vi "Kinect.vi"(8 "Right Right / Left 2":refnum<vi>, 9 "Right Up / Down 2":refnum<vi>, 10 "Left Right / Left 2":refnum<vi>, 11 "Left Up / Down 2":refnum<vi>) -> ()   [LabVIEW 2014]
doc: "Use this template to build a producer/consumer design pattern with events to produce queue items. Use this design pattern instead of the User Interface Event Handler pattern for user interfaces when you want to execute code asynchronously in response to an event without slowing the user interface responsiveness."
uses:
  System.Speech
  Kinect Library/Kinect Type Defs/Color Image Format.ctl
  Kinect Library/Kinect Type Defs/Depth Image Format.ctl
  Kinect Library/Kinect Session Class/Kinect Session.lvclass
  Kinect Library/Kinect Library.lvlib
panel:
  out "Start / Stop":bool
  out "Left Right / Left":sgl(slide) min=-0.5 max=0.5 scale=0.5..-0.5
  out "Right Right / Left":sgl(slide) min=-0.5 max=0.5 scale=-0.5..0.5
  out "Right Up / Down":sgl(slide) min=-0.5 max=0.5 scale=-0.5..0.5
  out "Left Up / Down":sgl(slide) min=-0.5 max=0.5 scale=-0.5..0.5
  out "Skeletal Data":T1(array[cluster])
  in  "Kinect\nVertical Angle\n[Enter]":i32(slide) min=-27 max=27 scale=-27.0..27.0
  out "Depth Frame":T2(plugin-control)
  out "Color Frame":T2(plugin-control)
  out "Status":string="Disconnected"
  in  "Disconnect Button":bool
  in  "Connect Kinect":bool
  in  "stop":bool
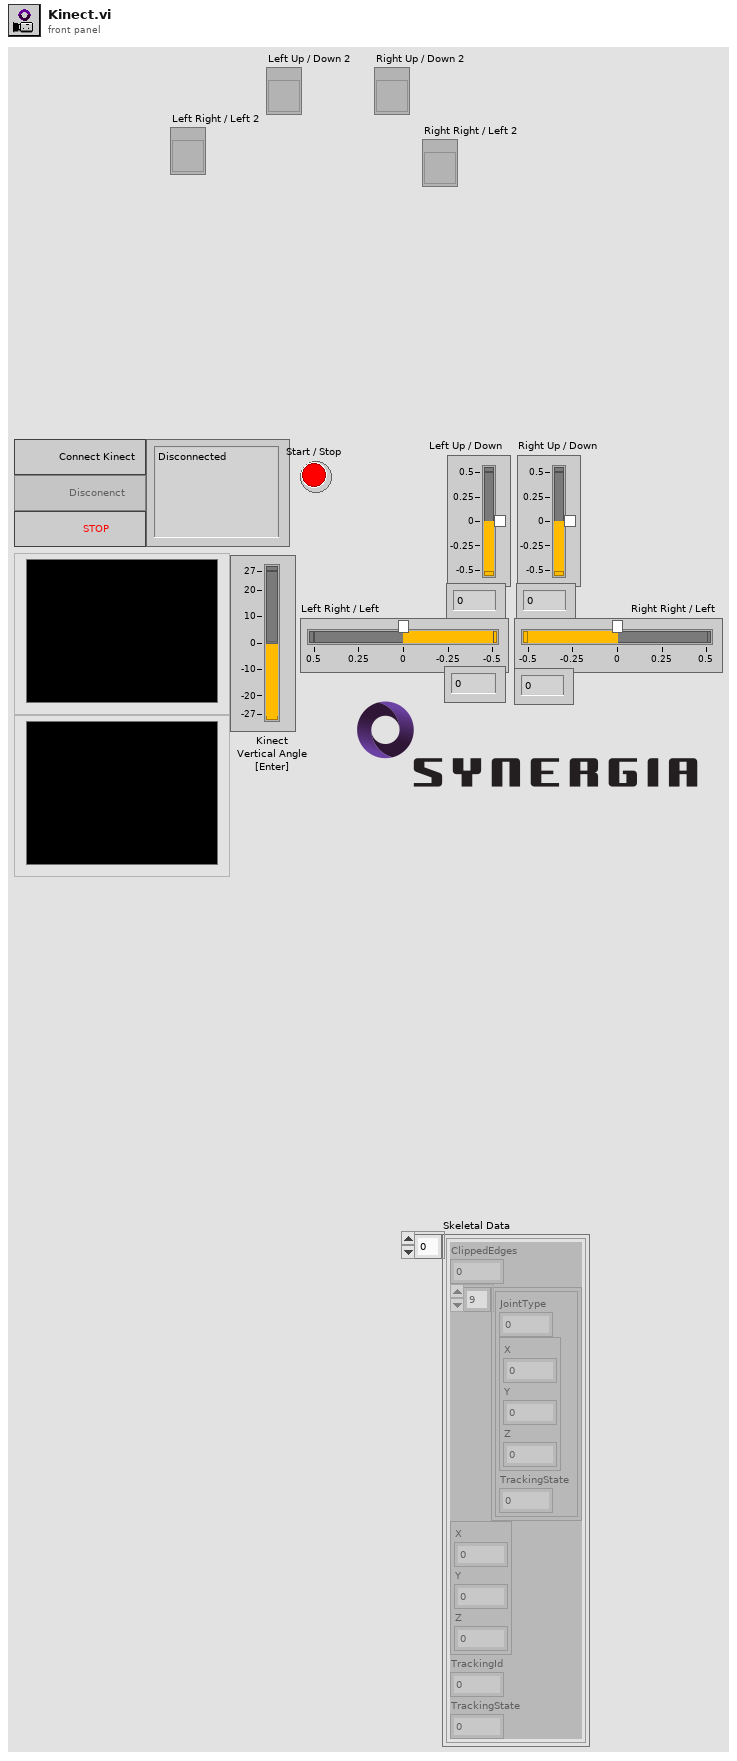
[diagram p1: front panel]
types:
  T1 = cluster{"ClippedEdges":i32, cluster{"JointType":i32, cluster{"X":sgl, "Y":sgl, "Z":sgl}, "TrackingState":i32}[], cluster{"X":sgl, "Y":sgl, "Z":sgl}, "TrackingId":i32, "TrackingState":i32}[]
  T2 = typedef "IMAQ Image.ctl" = refnum<image>
  T3 = enum8{"Enabled", "Disabled", "Disabled and Grayed Out"}
  T4 = typedef "Kinect Library.lvlib/Depth Image Format.ctl" = enum16{"Default", "Undefined", "Resolution640x480Fps30", "Resolution320x240Fps30", "Resolution80x60Fps30"}
  T5 = typedef "Kinect Library.lvlib/Color Image Format.ctl" = enum16{"Default", "Undefined", "RgbResolution640x480Fps30", "RgbResolution1280x960Fps12", "YuvResolution640x480Fps15", "RawYuvResolution640x480Fps15"}
  T6 = cluster{"ClippedEdges":i32, cluster{"JointType":i32, cluster{"X":sgl, "Y":sgl, "Z":sgl}, "TrackingState":i32}[], cluster{"X":sgl, "Y":sgl, "Z":sgl}, "TrackingId":i32, "TrackingState":i32}
  T7 = cluster{"JointType":i32, cluster{"X":sgl, "Y":sgl, "Z":sgl}, "TrackingState":i32}[]
  T8 = cluster{"JointType":i32, cluster{"X":sgl, "Y":sgl, "Z":sgl}, "TrackingState":i32}
  T9 = typedef "eventvkey.ctl" = enum16{"ASCII", "Enter", "Return", "Shift", "Ctrl", "Alt", "Cmd", "Opt", "Caps", "NumLock", "Clear", "Break", "Up", "Down", "Left", "Right", "Insert", "Delete", "Home", "End", "PageUp", "PageDown", "Escape", "Help", "Pause", "ScrollLock", "F1", "F2", "F3", "F4", "F5", "F6", "F7", "F8", "F9", "F10", "F11", "F12", "F13", "F14", "F15", "F16", "F17", "F18", "F19", "F20", "F21", "F22", "F23", "F24", "Play", "VolumeUp", "VolumeDown", "Mute", "Two Byte Char"}
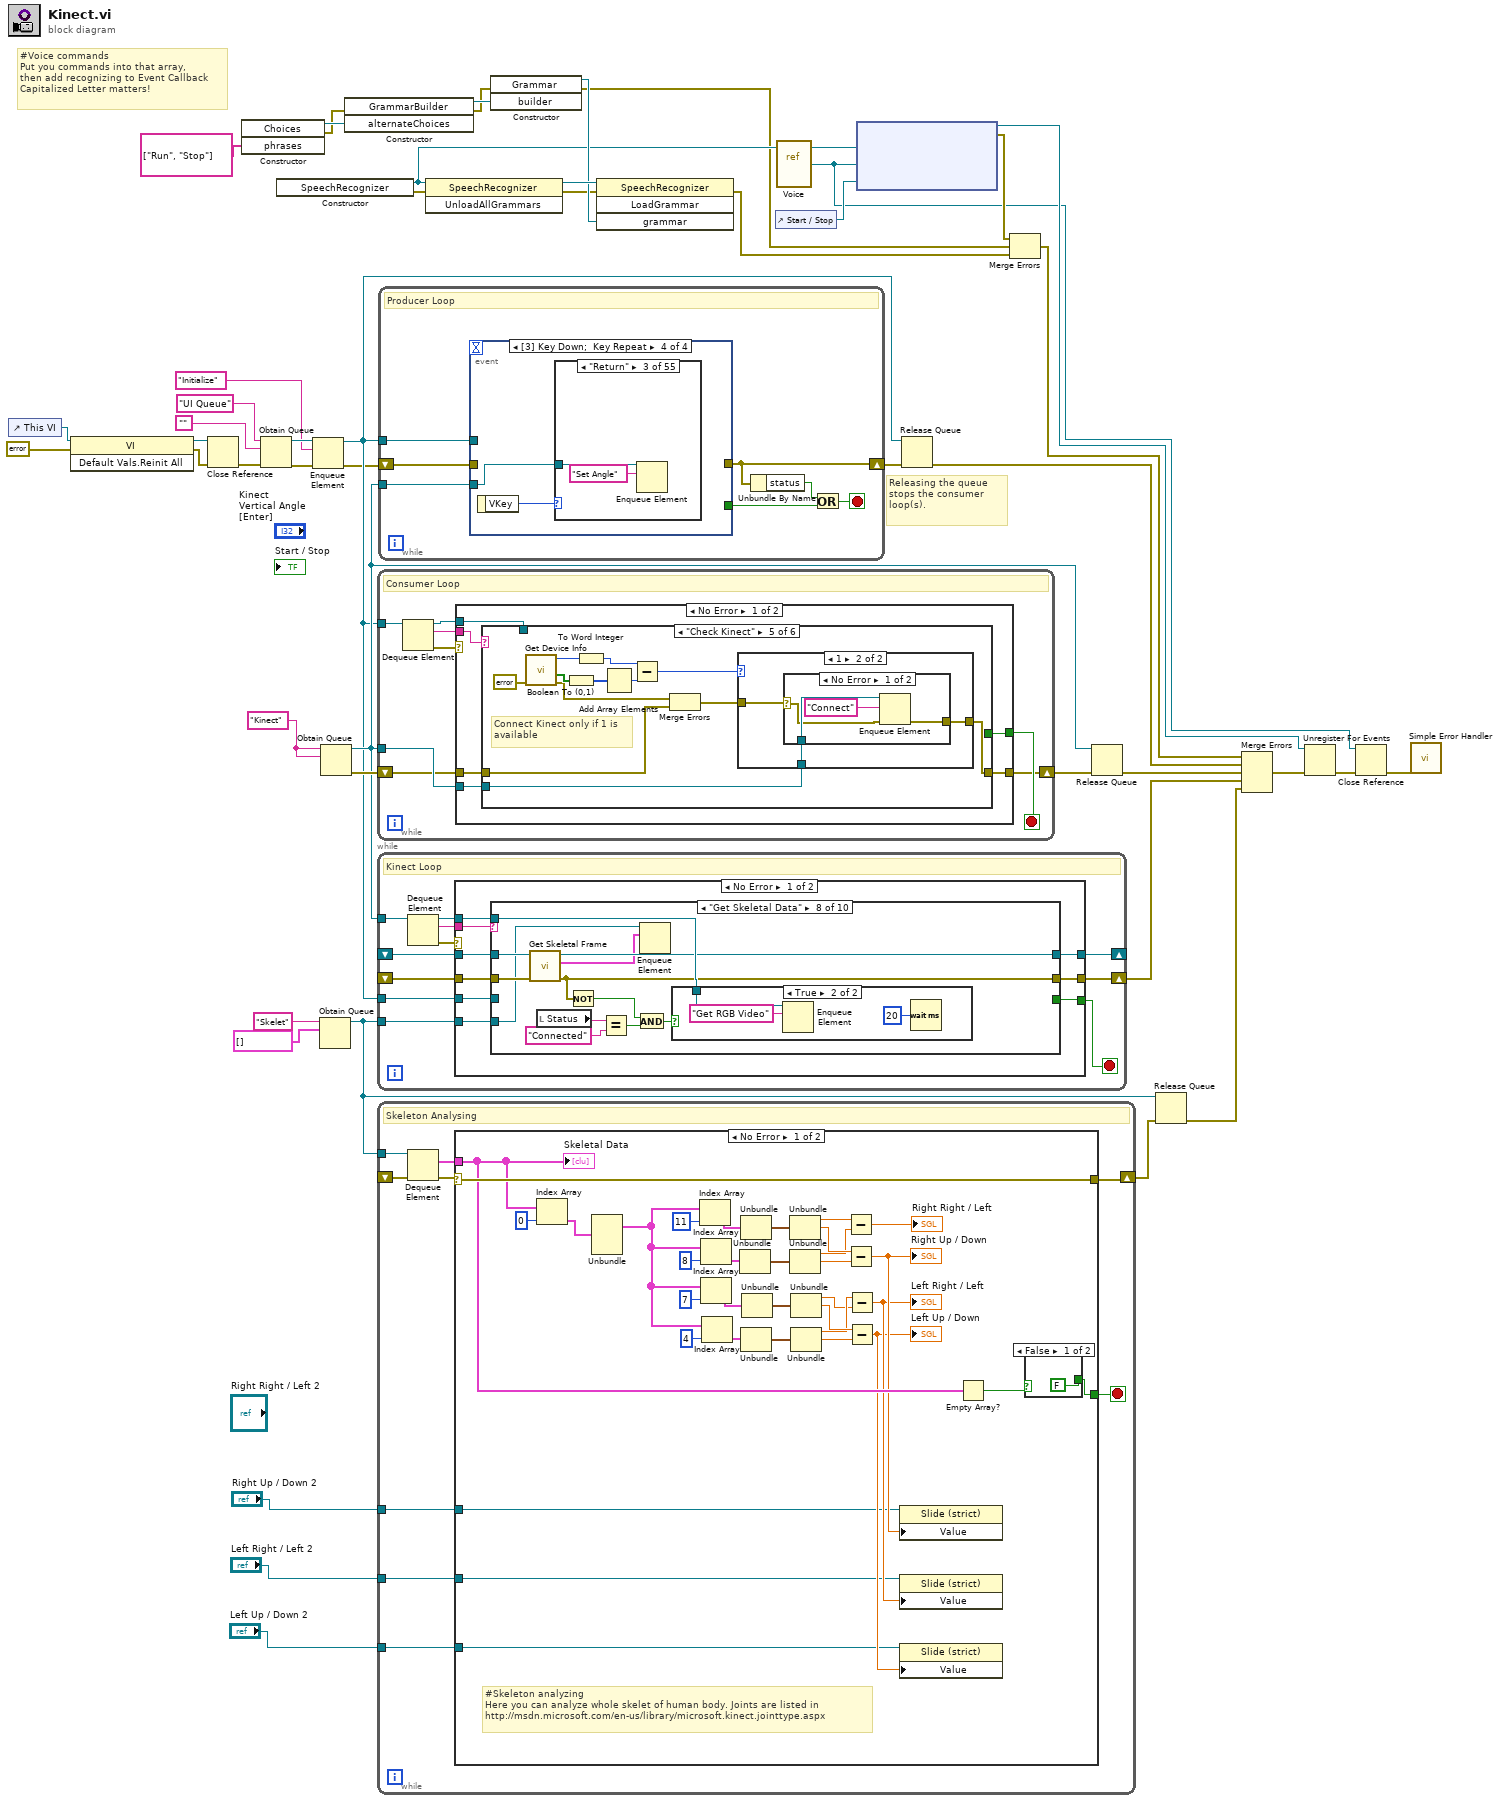
[diagram p0: block diagram]
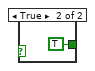
[diagram p2: hidden frame]
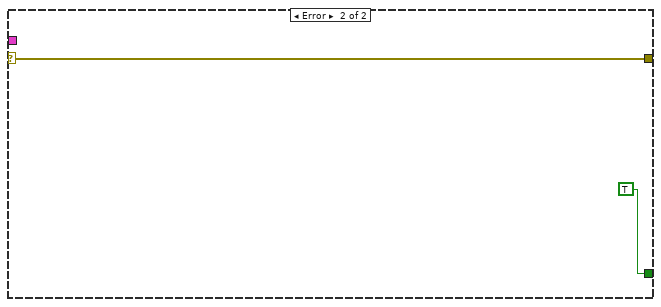
[diagram p3: hidden frame]
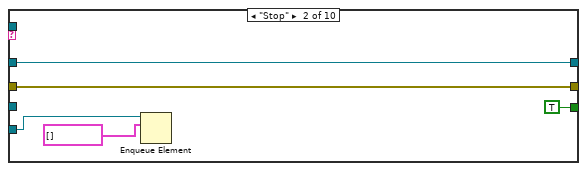
[diagram p5: hidden frame]
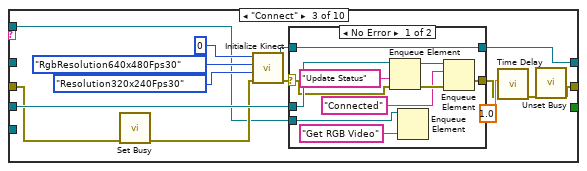
[diagram p6: hidden frame]
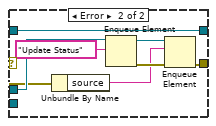
[diagram p7: hidden frame]
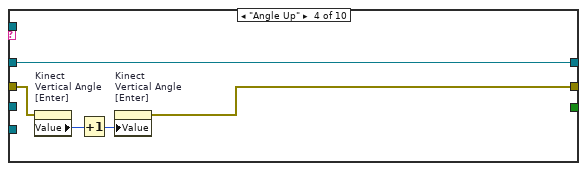
[diagram p8: hidden frame]
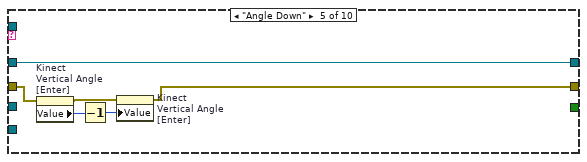
[diagram p9: hidden frame]
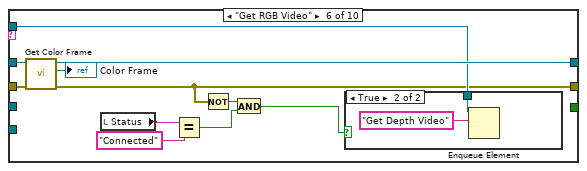
[diagram p10: hidden frame]
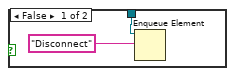
[diagram p11: hidden frame]
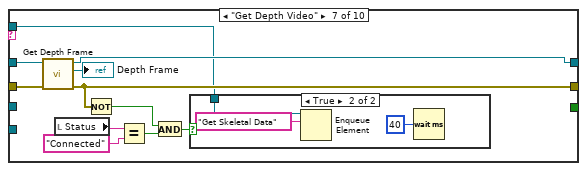
[diagram p12: hidden frame]
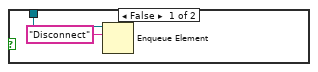
[diagram p13: hidden frame]
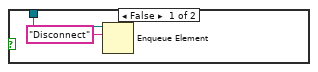
[diagram p14: hidden frame]
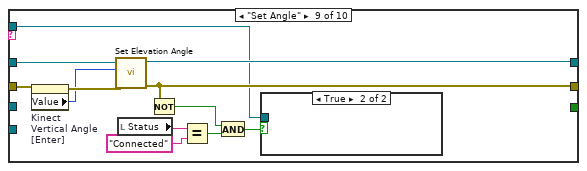
[diagram p15: hidden frame]
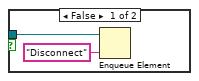
[diagram p16: hidden frame]
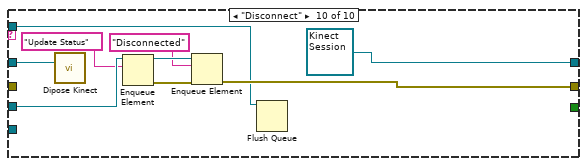
[diagram p17: hidden frame]
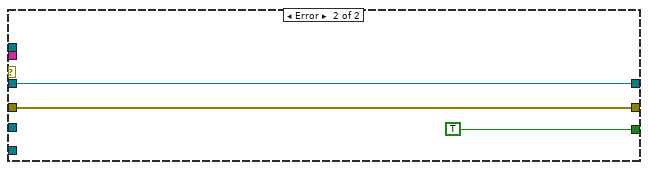
[diagram p18: hidden frame]
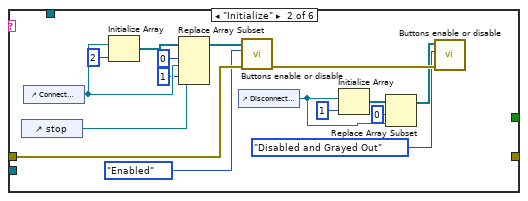
[diagram p20: hidden frame]
diagram:
  w38 = "Kinect" ("name (unnamed)")
  # "#Voice commands\nPut you commands into that array,\nthen add recognizing to Event Callback\nCapitalized Letter matters!"
  # "Releasing the queue stops the consumer loop(s)."
  n1 = control-ref of="This VI"() -> (w45:refnum<vi>)
  n2 = invoke class="VI" method="Default Vals.Reinit All"(reference=w45, error in=errorcluster {"status"=FALSE, "code"=0, "source"=""} ("error in (no error)")) -> (reference out=w44:refnum<vi>, error out=w43:errorcluster)  [unwired: 1 in, 1 out]
  n3 = Close Reference(reference=w44, error in (no error)=w43) -> (error out=w42:errorcluster)
  n4 = constructor class="Choices"("phrases"=string[] ["Run", "Stop"]) -> (reference out=w22:refnum<k24>, error out=w16:errorcluster)  [unwired: 3 in, 2 out]
  n5 = Obtain Queue(name (unnamed)="UI Queue", element data type="" ("data (can be any type)"), error in (no error)=w42) -> (queue out=w33:refnum<queue>, error out=w30:errorcluster)  [unwired: 2 in, 1 out]
  n6 = constructor class="SpeechRecognizer"() -> (reference out=w18:refnum<k24>, error out=w14:errorcluster)  [unwired: 3 in, 1 out]
  n7 = Enqueue Element(queue=w33, element="Initialize", error in (no error)=w30) -> (queue out=w32:refnum<queue>, error out=w31:errorcluster)  [unwired: 1 in, 1 out]
  n8 = Obtain Queue(name (unnamed)="Skelet", element data type=T1 [] ("Skeletal Data")) -> (queue out=w25:refnum<queue>)  [unwired: 3 in, 2 out]
  n9 = Obtain Queue(name (unnamed)=w38, element data type=w38) -> (queue out=w34:refnum<queue>, error out=w40:errorcluster)  [unwired: 3 in, 1 out]
  n10 = constructor class="GrammarBuilder"(error in=w16, "alternateChoices"=w22) -> (reference out=w21:refnum<k24>, error out=w15:errorcluster)  [unwired: 2 in, 2 out]
  n11 = while {
    tunnel: w32 -> [w56]
    shift-right: [w51] -> w39
    shift-left: w40 -> [w50]
    tunnel: w34 -> [w52]
    stop <- w53 stop-if-true
    # "Consumer Loop"
    n12 = Dequeue Element(queue=w56) -> (queue out=w49:refnum<queue>, element=w54:string, error out=w55:errorcluster)  [unwired: 2 in, 1 out]
    n13 = case shown="No Error" w55 {
      selector: w55 -> [_ w136]
      tunnel: w54 -> [w62 _]
      tunnel: [w57 TRUE] -> w53
      tunnel: w52 -> [w61 _]
      tunnel: [w60 w136] -> w51
      tunnel: w50 -> [w59 _]
      tunnel: w49 -> [w58 _]
      frame No Error {
        n14 = case shown="\"Check Kinect\"" w62 {
          tunnel: w61 -> [_ _ _ _ w113 w135]
          tunnel: [w63 _ w80 w82 w112 w132] -> w60
          tunnel: w59 -> [w63 w73 w80 w85 w110 w133]
          tunnel: w58 -> [_ _ _ w87 _ _]
          tunnel: [_ _ TRUE _ _ _] -> w57
          frame Default {
          }
          frame "Initialize" {
            n15 = control-ref of="stop"() -> (w74:refnum<vi>)
            n16 = control-ref of="Connect Kinect"() -> (w76:refnum<vi>)
            n17 = Initialize Array(w76, 2 ("dimension size")) -> (w78:refnum<vi>[])
            n18 = Replace Array Subset(array=w78, new element #1=w76, index #1=0 ("index"), new element #2=w74, index #2=1 ("index")) -> (w72:refnum<vi>[])
            n19 = control-ref of="Disconnect Button"() -> (w66:refnum<vi>)
            n20 = call "Buttons enable or disable.vi"("error in (no error)"=w73, "Enabled or Disabled?"=T3."Enabled", "Input references array"=w72) -> ("error out"=w70:errorcluster)  [unwired: 8 in]
            n21 = Initialize Array(w66, 1 ("dimension size")) -> (w68:refnum<vi>[])
            n22 = Replace Array Subset(array=w68, new element=w66, index=0) -> (w65:refnum<vi>[])
            n23 = call "Buttons enable or disable.vi"("error in (no error)"=w70, "Enabled or Disabled?"=T3."Disabled and Grayed Out", "Input references array"=w65) -> ()  [unwired: 8 in, 1 out]
          }
          frame "Stop" {
          }
          frame "Update Status" {
            n24 = Dequeue Element(queue=w87) -> (element=w84:string, error out=w86:errorcluster)  [unwired: 2 in, 2 out]
            "Status" <- w84
            n25 = Merge Errors(w86, w85) -> (w83:errorcluster)
            n26 = case shown="\"Disconnected\"" w84 {
              tunnel: w83 -> [w88 w96 w108]
              tunnel: [w88 w90 w99] -> w82
              frame Default {
              }
              frame "Connected" {
                n27 = control-ref of="Disconnect Button"() -> (w98:refnum<vi>)
                n28 = Build Array(w98) -> (w97:refnum<vi>[])
                n29 = call "Buttons enable or disable.vi"("error in (no error)"=w96, "Enabled or Disabled?"=T3."Enabled", "Input references array"=w97) -> ("error out"=w91:errorcluster)  [unwired: 8 in]
                n30 = control-ref of="stop"() -> (w93:refnum<vi>)
                n31 = control-ref of="Connect Kinect"() -> (w92:refnum<vi>)
                n32 = Build Array(w93, w92) -> (w94:refnum<vi>[])
                n33 = call "Buttons enable or disable.vi"("error in (no error)"=w91, "Enabled or Disabled?"=T3."Disabled and Grayed Out", "Input references array"=w94) -> ("error out"=w90:errorcluster)  [unwired: 8 in]
              }
              frame "Disconnected" {
                n34 = control-ref of="Disconnect Button"() -> (w107:refnum<vi>)
                n35 = Build Array(w107) -> (w106:refnum<vi>[])
                n36 = call "Buttons enable or disable.vi"("error in (no error)"=w108, "Enabled or Disabled?"=T3."Disabled and Grayed Out", "Input references array"=w106) -> ("error out"=w101:errorcluster)  [unwired: 8 in]
                n37 = control-ref of="Connect Kinect"() -> (w103:refnum<vi>)
                n38 = control-ref of="stop"() -> (w102:refnum<vi>)
                n39 = Build Array(w103, w102) -> (w104:refnum<vi>[])
                n40 = call "Buttons enable or disable.vi"("error in (no error)"=w101, "Enabled or Disabled?"=T3."Enabled", "Input references array"=w104) -> ("error out"=w99:errorcluster)  [unwired: 8 in]
              }
            }
          }
          frame "Check Kinect" {
            # "Connect Kinect only if 1 is\navailable"
            n41 = call "Get Device Info.vi"("error in (no error)"=errorcluster {"status"=FALSE, "code"=0, "source"=""}) -> ("error out"=w111:errorcluster, "Is Running"=w119:bool[], "Number of Kinects Attached"=w116:i32)  [unwired: 7 in, 1 out]
            n42 = Boolean To (0,1)(Boolean=w119) -> (0, 1=w118:i16[])
            n43 = To Word Integer(number=w116) -> (16bit integer=w115:i16)
            n44 = Add Array Elements(numeric array=w118) -> (sum=w117:i16)
            n45 = Subtract(x=w115, y=w117) -> (x-y=w114:i16)
            n46 = Merge Errors(w111, w110) -> (w109:errorcluster)
            n47 = case shown="1" w114 {
              tunnel: w109 -> [w122 w124]
              tunnel: w113 -> [_ w125]
              tunnel: [w121 w123] -> w112
              frame 0, Default {
                n48 = call "Display Message to User"("error in (no error)"=w122) -> ("error out"=w121:errorcluster)  [unwired: 9 in, 1 out]
              }
              frame 1 {
                n49 = case shown="No Error" w124 {
                  selector: w124 -> [w127 w131]
                  tunnel: w125 -> [w129 _]
                  tunnel: [w126 w130] -> w123
                  frame No Error {
                    n50 = Enqueue Element(queue=w129, element="Connect", error in (no error)=w127) -> (error out=w126:errorcluster)  [unwired: 1 in, 2 out]
                  }
                  frame Error {
                    n51 = call "Display Message to User2"("error in (no error)"=w131) -> ("error out"=w130:errorcluster)  [unwired: 9 in, 1 out]
                  }
                }
              }
            }
          }
          frame "Disconnect Kinect" {
            n52 = Enqueue Element(queue=w135, element="Disconnect", error in (no error)=w133) -> (error out=w132:errorcluster)  [unwired: 1 in, 2 out]
          }
        }
      }
      frame Error {
        # "Return true in any case that should stop the loop."
      }
    }
  }
  n53 = while {
    tunnel: w34 -> [w148]
    shift-right: [w144] -> _
    shift-left: _ -> [w143]
    shift-right: [w142] -> w35
    shift-left: _ -> [w141]
    tunnel: w32 -> [w140]
    tunnel: w25 -> [w138]
    stop <- w139 stop-if-true
    # "Kinect Loop"
    n54 = Dequeue Element(queue=w148) -> (queue out=w146:refnum<queue>, element=w145:string, error out=w147:errorcluster)  [unwired: 2 in, 1 out]
    n55 = case shown="No Error" w147 {
      tunnel: w146 -> [w151 _]
      tunnel: w145 -> [w157 _]
      tunnel: [w150 TRUE] -> w139
      tunnel: [w156 w280] -> w144
      tunnel: w143 -> [w155 w280]
      tunnel: [w154 w279] -> w142
      tunnel: w141 -> [w153 w279]
      tunnel: w140 -> [w152 _]
      tunnel: w138 -> [w149 _]
      frame No Error {
        n56 = case shown="\"Get Skeletal Data\"" w157 {
          tunnel: [w159 w162 w173 w197 w202 w216 w230 w241 w266 refnum<class "Kinect Session.lvclass"> refnum ("Kinect Session out")] -> w156
          tunnel: w155 -> [w159 w162 _ w197 w202 w218 w233 w242 w267 w277]
          tunnel: [w158 w163 w166 w198 w203 w208 w229 w243 w258 w271] -> w154
          tunnel: w153 -> [w158 w163 w172 w200 w207 w217 w232 w244 w265 _]
          tunnel: w152 -> [_ _ w175 _ _ _ _ _ _ w276]
          tunnel: w151 -> [_ _ w169 _ _ w211 w223 w245 w256 w270]
          tunnel: [_ TRUE _ _ _ _ _ _ _ _] -> w150
          tunnel: w149 -> [_ w161 _ _ _ _ _ w240 _ _]
          frame Default {
          }
          frame "Stop" {
            n57 = Enqueue Element(queue=w161, element=T1 [] ("Skeletal Data")) -> ()  [unwired: 2 in, 3 out]
          }
          frame "Connect" {
            n58 = call <vilib>:"Set Busy.vi"("error in (no error)"=w172) -> ("error out"=w171:errorcluster)  [unwired: 9 in, 1 out]
            n59 = call "Initialize Kinect.vi"("error in (no error)"=w171, "Depth Image Format"=Depth_Image_Format."Resolution320x240Fps30", "Color Image Format"=Color_Image_Format."RgbResolution640x480Fps30", "Kinect Sensor Index"=0) -> ("error out"=w170:errorcluster, "Kinect Session out"=w174:refnum<class "Kinect Session.lvclass">)  [unwired: 6 in]
            n60 = case shown="No Error" w170 {
              selector: w170 -> [w186 w191]
              tunnel: w175 -> [w188 w196]
              tunnel: w174 -> [w181 w189]
              tunnel: [w184 w193] -> w165
              tunnel: [w181 w189] -> w173
              tunnel: w169 -> [w180 _]
              frame No Error {
                n61 = Enqueue Element(queue=w188, element="Update Status", error in (no error)=w186) -> (queue out=w182:refnum<queue>, error out=w185:errorcluster)  [unwired: 1 in, 1 out]
                n62 = Enqueue Element(queue=w180, element="Get RGB Video") -> ()  [unwired: 2 in, 3 out]
                n63 = Enqueue Element(queue=w182, element="Connected", error in (no error)=w185) -> (error out=w184:errorcluster)  [unwired: 1 in, 2 out]
              }
              frame Error {
                n64 = Unbundle By Name(w191) -> ("source"=w190:string)
                n65 = Enqueue Element(queue=w196, element="Update Status") -> (queue out=w194:refnum<queue>, error out=w192:errorcluster)  [unwired: 2 in, 1 out]
                n66 = Enqueue Element(queue=w194, element=w190, error in (no error)=w192) -> (error out=w193:errorcluster)  [unwired: 1 in, 2 out]
              }
            }
            n67 = call "Time Delay"("error in (no error)"=w165, "Delay Time (s)"=1.0) -> ("error out"=w167:errorcluster)  [unwired: 9 in]
            n68 = call <vilib>:"Unset Busy.vi"("error in (no error)"=w167) -> ("error out"=w166:errorcluster)  [unwired: 10 in]
          }
          frame "Angle Up" {
            n69 = property on="Kinect\nVertical Angle\n[Enter]" class="Slide (strict)"(error in=w200) -> ("Value"=w201:i32)  [unwired: 1 in, 2 out]
            n70 = Increment(x=w201) -> (x+1=w199:i32)
            n71 = property on="Kinect\nVertical Angle\n[Enter]" class="Slide (strict)"("Value"=w199) -> (error out=w198:errorcluster)  [unwired: 2 in, 1 out]
          }
          frame "Angle Down" {
            n72 = property on="Kinect\nVertical Angle\n[Enter]" class="Slide (strict)"(error in=w207) -> (error out=w205:errorcluster, "Value"=w206:i32)  [unwired: 1 in, 1 out]
            n73 = Decrement(x=w206) -> (x-1=w204:i32)
            n74 = property on="Kinect\nVertical Angle\n[Enter]" class="Slide (strict)"(error in=w205, "Value"=w204) -> (error out=w203:errorcluster)  [unwired: 1 in, 1 out]
          }
          frame "Get RGB Video" {
            n75 = call "Get Color Frame.vi"("error in (no error)"=w217, "Kinect Session in"=w218) -> ("error out"=w208:errorcluster, "Color Frame"=→"Color Frame":T2, "Kinect Session out"=w216:refnum<class "Kinect Session.lvclass">)  [unwired: 7 in]
            n76 = local read "Status"() -> (w214:string)
            n77 = Equal?(x=w214, y="Connected") -> (x = y?=w209:bool)
            n78 = Not(x=w208) -> (.not. x?=w210:bool)
            n79 = And(x=w210, y=w209) -> (x .and. y?=w212:bool)
            n80 = case shown="True" w212 {
              tunnel: w211 -> [w220 w222]
              frame False {
                n81 = Enqueue Element(queue=w220, element="Disconnect") -> ()  [unwired: 2 in, 3 out]
              }
              frame True {
                n82 = Enqueue Element(queue=w222, element="Get Depth Video") -> ()  [unwired: 2 in, 3 out]
              }
            }
          }
          frame "Get Depth Video" {
            n83 = call "Get Depth Frame.vi"("error in (no error)"=w232, "Kinect Session in"=w233) -> ("error out"=w229:errorcluster, "Depth Frame"=→"Depth Frame":T2, "Kinect Session out"=w230:refnum<class "Kinect Session.lvclass">)  [unwired: 7 in]
            n84 = local read "Status"() -> (w228:string)
            n85 = Not(x=w229) -> (.not. x?=w225:bool)
            n86 = Equal?(x=w228, y="Connected") -> (x = y?=w226:bool)
            n87 = And(x=w225, y=w226) -> (x .and. y?=w224:bool)
            n88 = case shown="True" w224 {
              tunnel: w223 -> [w235 w238]
              frame False {
                n89 = Enqueue Element(queue=w235, element="Disconnect") -> ()  [unwired: 2 in, 3 out]
              }
              frame True {
                n90 = Enqueue Element(queue=w238, element="Get Skeletal Data") -> ()  [unwired: 2 in, 3 out]
                n91 = Wait (ms)(milliseconds to wait=u32 40) -> ()  [unwired: 1 out]
              }
            }
          }
          frame "Get Skeletal Data" {
            n92 = call "Get Skeletal Frame.vi"("error in (no error)"=w244, "Kinect Session in"=w242) -> ("error out"=w243:errorcluster, "Skeletal Data"=w239:T1, "Kinect Session out"=w241:refnum<class "Kinect Session.lvclass">)  [unwired: 7 in]
            n93 = local read "Status"() -> (w250:string)
            n94 = Not(x=w243) -> (.not. x?=w247:bool)
            n95 = Equal?(x=w250, y="Connected") -> (x = y?=w248:bool)
            n96 = And(x=w247, y=w248) -> (x .and. y?=w246:bool)
            n97 = Enqueue Element(queue=w240, element=w239) -> ()  [unwired: 2 in, 3 out]
            n98 = case shown="True" w246 {
              tunnel: w245 -> [w252 w255]
              frame False {
                n99 = Enqueue Element(queue=w252, element="Disconnect") -> ()  [unwired: 2 in, 3 out]
              }
              frame True {
                n100 = Enqueue Element(queue=w255, element="Get RGB Video") -> ()  [unwired: 2 in, 3 out]
                n101 = Wait (ms)(milliseconds to wait=u32 20) -> ()  [unwired: 1 out]
              }
            }
          }
          frame "Set Angle" {
            n102 = property on="Kinect\nVertical Angle\n[Enter]" class="Slide (strict)"(error in=w265) -> (error out=w264:errorcluster, "Value"=w263:i32)  [unwired: 1 in, 1 out]
            n103 = call "Set Elevation Angle.vi"("error in (no error)"=w264, "ElevationAngle"=w263, "Kinect Session in"=w267) -> ("error out"=w258:errorcluster, "Kinect Session out"=w266:refnum<class "Kinect Session.lvclass">)  [unwired: 6 in, 1 out]
            n104 = local read "Status"() -> (w262:string)
            n105 = Not(x=w258) -> (.not. x?=w259:bool)
            n106 = Equal?(x=w262, y="Connected") -> (x = y?=w260:bool)
            n107 = And(x=w259, y=w260) -> (x .and. y?=w257:bool)
            n108 = case shown="True" w257 {
              tunnel: w256 -> [w269 _]
              frame False {
                n109 = Enqueue Element(queue=w269, element="Disconnect") -> ()  [unwired: 2 in, 3 out]
              }
              frame True {
              }
            }
          }
          frame "Disconnect" {
            n110 = call "Dipose Kinect.vi"("Kinect Session in"=w277) -> ()  [unwired: 10 in, 1 out]
            n111 = Enqueue Element(queue=w276, element="Update Status") -> (queue out=w274:refnum<queue>, error out=w272:errorcluster)  [unwired: 2 in, 1 out]
            n112 = Enqueue Element(queue=w274, element="Disconnected", error in (no error)=w272) -> (error out=w271:errorcluster)  [unwired: 1 in, 2 out]
            n113 = Flush Queue(queue=w270) -> ()  [unwired: 1 in, 3 out]
          }
        }
      }
      frame Error {
      }
    }
  }
  n114 = while {
    tunnel: w25 -> [w290]
    shift-right: [w285] -> w24
    shift-left: _ -> [w286]
    tunnel: "Left Up / Down 2" -> [w284]
    tunnel: "Left Right / Left 2" -> [w283]
    tunnel: "Right Up / Down 2" -> [w282]
    stop <- w288 stop-if-true
    # "Skeleton Analysing"
    n115 = Dequeue Element(queue=w290, error in (no error)=w286) -> (element=w287:T1, error out=w289:errorcluster)  [unwired: 1 in, 2 out]
    n116 = case shown="No Error" w289 {
      selector: w289 -> [w324 w327]
      tunnel: [w322 TRUE] -> w288
      tunnel: w287 -> [w321 _]
      tunnel: [w324 w327] -> w285
      tunnel: w284 -> [w293 _]
      tunnel: w283 -> [w292 _]
      tunnel: w282 -> [w291 _]
      frame No Error {
        # "#Skeleton analyzing\nHere you can analyze whole skelet of human body. Joints are listed in\nhttp://msdn.microsoft.com/en-us/library/microsoft.kinect.jointtype.aspx"
        n117 = Index Array(array=w321, index=0) -> (element=w319:T6)
        n118 = Unbundle(w319) -> (w300:T7)  [unwired: 4 out]
        n119 = Index Array(array=w300, index=11) -> (element=w316:T8)
        n120 = Index Array(array=w300, index=8) -> (element=w315:T8)
        n121 = Index Array(array=w300, index=7) -> (element=w303:T8)
        n122 = Index Array(array=w300, index=4) -> (element=w304:T8)
        n123 = Unbundle(w315) -> (w313:cluster{"X":sgl, "Y":sgl, "Z":sgl})  [unwired: 2 out]
        n124 = Unbundle(w316) -> (w314:cluster{"X":sgl, "Y":sgl, "Z":sgl})  [unwired: 2 out]
        n125 = Unbundle(w304) -> (w306:cluster{"X":sgl, "Y":sgl, "Z":sgl})  [unwired: 2 out]
        n126 = Unbundle(w303) -> (w305:cluster{"X":sgl, "Y":sgl, "Z":sgl})  [unwired: 2 out]
        n127 = Unbundle(w314) -> ("X"=w310:sgl, "Y"=w312:sgl)  [unwired: 1 out]
        n128 = Unbundle(w313) -> ("X"=w309:sgl, "Y"=w311:sgl)  [unwired: 1 out]
        n129 = Unbundle(w305) -> ("X"=w298:sgl, "Y"=w307:sgl)  [unwired: 1 out]
        n130 = Unbundle(w306) -> ("X"=w299:sgl, "Y"=w308:sgl)  [unwired: 1 out]
        n131 = Subtract(x=w310, y=w309) -> (x-y=→"Right Right / Left":sgl)
        n132 = Subtract(x=w312, y=w311) -> (x-y=w296:sgl)
        "Right Up / Down" <- w296
        n133 = Subtract(x=w299, y=w298) -> (x-y=w295:sgl)
        "Left Right / Left" <- w295
        n134 = Subtract(x=w307, y=w308) -> (x-y=w294:sgl)
        "Left Up / Down" <- w294
        n135 = property class="Slide (strict)"(reference=w291, "Value"=w296) -> ()  [unwired: 1 in, 2 out]
        n136 = property class="Slide (strict)"(reference=w292, "Value"=w295) -> ()  [unwired: 1 in, 2 out]
        n137 = property class="Slide (strict)"(reference=w293, "Value"=w294) -> ()  [unwired: 1 in, 2 out]
        n138 = Empty Array?(array=w321) -> (empty?=w323:bool)
        n139 = case shown="False" w323 {
          tunnel: [FALSE TRUE] -> w322
          frame False {
          }
          frame True {
          }
        }
        "Skeletal Data" <- w321
      }
      frame Error {
      }
    }
  }
  n140 = while {
    shift-right: [w331] -> w48
    shift-left: w31 -> [w334]
    tunnel: w32 -> [w335]
    tunnel: w34 -> [w329]
    stop <- w332 stop-if-true
    # "Producer Loop"
    n141 = event shown="[3] Key Down;  Key Repeat" {
      selector: _ -> [_ _ _ _]
      dyn-events: _ -> [_ _ _ _]
      timeout: _ -> [_ _ _ _]
      tunnel: w335 -> [w339 w345 w347 _]
      tunnel: w334 -> [w340 w343 w349 _]
      tunnel: [w340 w342 w348 _] -> w331
      tunnel: ["stop" _ _ _] -> w333
      tunnel: w329 -> [w337 _ _ w350]
      event "stop": Value Change {
        n142 = event-data() -> ()  [unwired: 1 in, 1 out]
        n143 = Enqueue Element(queue=w339, element="Stop") -> ()  [unwired: 2 in, 3 out]
        n144 = Enqueue Element(queue=w337, element="Stop") -> ()  [unwired: 2 in, 3 out]
      }
      event "Connect Kinect": Value Change {
        n145 = event-data() -> ()  [unwired: 1 in, 1 out]
        n146 = Enqueue Element(queue=w345, element="Check Kinect", error in (no error)=w343) -> (error out=w342:errorcluster)  [unwired: 1 in, 2 out]
      }
      event "Disconnect Button": Value Change {
        n147 = event-data() -> ()  [unwired: 1 in, 1 out]
        n148 = Enqueue Element(queue=w347, element="Disconnect Kinect", error in (no error)=w349) -> (error out=w348:errorcluster)  [unwired: 1 in, 2 out]
      }
      event Key Down; Key Repeat {
        n149 = event-data() -> ("VKey"=w351:T9)  [unwired: 1 in]
        n150 = case shown="\"Return\"" w351 {
          tunnel: w350 -> [_ _ w353 w355 w356 _ _ _ _ _ _ _ _ _ _ _ _ _ _ _ _ _ _ _ _ _ _ _ _ _ _ _ _ _ _ _ _ _ _ _ _ _ _ _ _ _ _ _ _ _ _ _ _ _ _]
          frame "ASCII", Default {
          }
          frame "Enter" {
          }
          frame "Return" {
            n151 = Enqueue Element(queue=w353, element="Set Angle") -> ()  [unwired: 2 in, 3 out]
          }
          frame "Shift" {
            n152 = Enqueue Element(queue=w355, element="Angle Up") -> ()  [unwired: 2 in, 3 out]
          }
          frame "Ctrl" {
            n153 = Enqueue Element(queue=w356, element="Angle Down") -> ()  [unwired: 2 in, 3 out]
          }
          frame "Alt" {
          }
          frame "Cmd" {
          }
          frame "Opt" {
          }
          frame "Caps" {
          }
          frame "NumLock" {
          }
          frame "Clear" {
          }
          frame "Break" {
          }
          frame "Up" {
          }
          frame "Down" {
          }
          frame "Left" {
          }
          frame "Right" {
          }
          frame "Insert" {
          }
          frame "Delete" {
          }
          frame "Home" {
          }
          frame "End" {
          }
          frame "PageUp" {
          }
          frame "PageDown" {
          }
          frame "Escape" {
          }
          frame "Help" {
          }
          frame "Pause" {
          }
          frame "ScrollLock" {
          }
          frame "F1" {
          }
          frame "F2" {
          }
          frame "F3" {
          }
          frame "F4" {
          }
          frame "F5" {
          }
          frame "F6" {
          }
          frame "F7" {
          }
          frame "F8" {
          }
          frame "F9" {
          }
          frame "F10" {
          }
          frame "F11" {
          }
          frame "F12" {
          }
          frame "F13" {
          }
          frame "F14" {
          }
          frame "F15" {
          }
          frame "F16" {
          }
          frame "F17" {
          }
          frame "F18" {
          }
          frame "F19" {
          }
          frame "F20" {
          }
          frame "F21" {
          }
          frame "F22" {
          }
          frame "F23" {
          }
          frame "F24" {
          }
          frame "Play" {
          }
          frame "VolumeUp" {
          }
          frame "VolumeDown" {
          }
          frame "Mute" {
          }
          frame "Two Byte Char" {
          }
        }
      }
    }
    n154 = Unbundle By Name(w331) -> ("status"=w330:bool)
    n155 = Or(x=w330, y=w333) -> (x .or. y?=w332:bool)
  }
  n156 = invoke class="SpeechRecognizer" method="UnloadAllGrammars"(reference=w18, error in=w14) -> (reference out=w20:refnum<k24>, error out=w13:errorcluster)  [unwired: 1 in, 1 out]
  n157 = constructor class="Grammar"(error in=w15, "builder"=w21) -> (reference out=w19:refnum<k24>, error out=w11:errorcluster)  [unwired: 2 in, 2 out]
  n158 = invoke class="SpeechRecognizer" method="LoadGrammar"(reference=w20, error in=w13, "grammar"=w19) -> (error out=w10:errorcluster)  [unwired: 1 in, 3 out]
  n159 = control-ref of="Start / Stop"() -> (w17:refnum<vi>)
  n160 = vi-ref "Voice.vi"() -> ("vi reference"=w6:refnum<vi>)
  n161 = node(w18, w6, w17) -> (w7:refnum<k27>, w12:errorcluster)  [unwired: 2 in]
  n162 = Release Queue(queue=w32, error in (no error)=w48) -> (error out=w37:errorcluster)  [unwired: 1 in, 2 out]
  n163 = Merge Errors(w12, w11, w10) -> (w9:errorcluster)
  n164 = Release Queue(queue=w34, error in (no error)=w39) -> (error out=w36:errorcluster)  [unwired: 1 in, 2 out]
  n165 = Release Queue(queue=w25, error in (no error)=w24) -> (error out=w27:errorcluster)  [unwired: 1 in, 2 out]
  n166 = Merge Errors(w9, w37, w36, w35, w27) -> (w5:errorcluster)
  n167 = Unregister For Events(event registration refnum=w7, error in=w5) -> (error out=w8:errorcluster)
  n168 = Close Reference(reference=w6, error in (no error)=w8) -> (error out=w4:errorcluster)
  n169 = call <vilib>:"Simple Error Handler.vi"("error in (no error)"=w4) -> ()  [unwired: 4 in, 5 out]
